vi "Start Search Params.vi"(8 "error in (no error)":errorcluster, 10 "Search in":refnum<class "Search.lvclass">, 11 "BetterSearch in":refnum<class "BetterSearch.lvclass">) -> (0 "error out":errorcluster, 2 "Start Params":T1, 3 "BetterSearch out":refnum<class "BetterSearch.lvclass">)   [LabVIEW 2020, in "Better Search.lvlib" / "BetterSearch.lvclass"]
uses:
  BetterSearch.lvclass
  Data Types/Search Params.ctl
  Data Types/Search Type.ctl
  Data Types/Search Scope.ctl
  Data Types/Scope Options.ctl
  Search/Search.lvclass
  BetterSearch.lvclass/BetterSearch.ctl
  Better Search.lvlib
panel:
  # "Exclude"
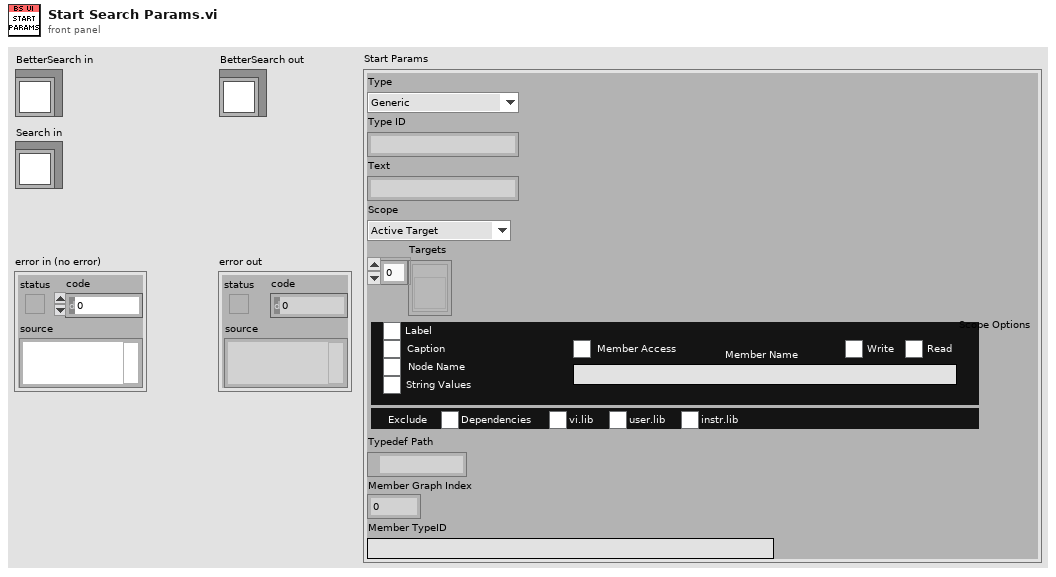
[diagram p1: front panel]
types:
  T1 = typedef "Better Search.lvlib/Search Params.ctl" = cluster{"Type":T2, "Type ID":string, "Text":string, "Scope":T3, "Targets":refnum<vi>[], "Scope Options":T4, "Typedef Path":path, "Member Graph Index":i32, "Member TypeID":string}
  T2 = typedef "Better Search.lvlib/Search Type.ctl" = enum16{"Generic", "Text", "Data Type", "VI", "Node"}
  T3 = typedef "Better Search.lvlib/Search Scope.ctl" = enum16{"Active Target", "Active Project", "Specific Targets", "Active VI", "Active Hierarchy"}
  T4 = typedef "Better Search.lvlib/Scope Options.ctl" = cluster{"Include Labels":bool, "Include Captions":bool, "Include Node Name":bool, "Member Access":bool, "Member Read":bool, "Member Write":bool, "Member Name":string, "String Value":bool, "Dependencies":bool, "vi.lib":bool, "user.lib":bool, "instr.lib":bool}
  T5 = typedef "Better Search.lvlib/Search Context.ctl" = cluster{"Type ID":string, "VI Refnum":refnum<vi>, "Starting Text":string, "Shift?":bool, "App Ref":refnum<vi>, "Start Search Type":T6, "Item Graph":T7[], "Variant":variant}
  T6 = typedef "Better Search.lvlib/Start Search Type.ctl" = enum16{"Auto", "Text", "Data Type", "Bundle"}
  T7 = typedef "Better Search.lvlib/Type Reflection Item.ctl" = cluster{"Parent":i32, "Depth":i32, "Children":i32[], "Skip":bool, "Name":string, "Type":variant, "TypeID":string}
  T8 = typedef "Better Search.lvlib/Search Type Info.ctl" = cluster{"Search Type":T2, "Name":string, "Item":variant}
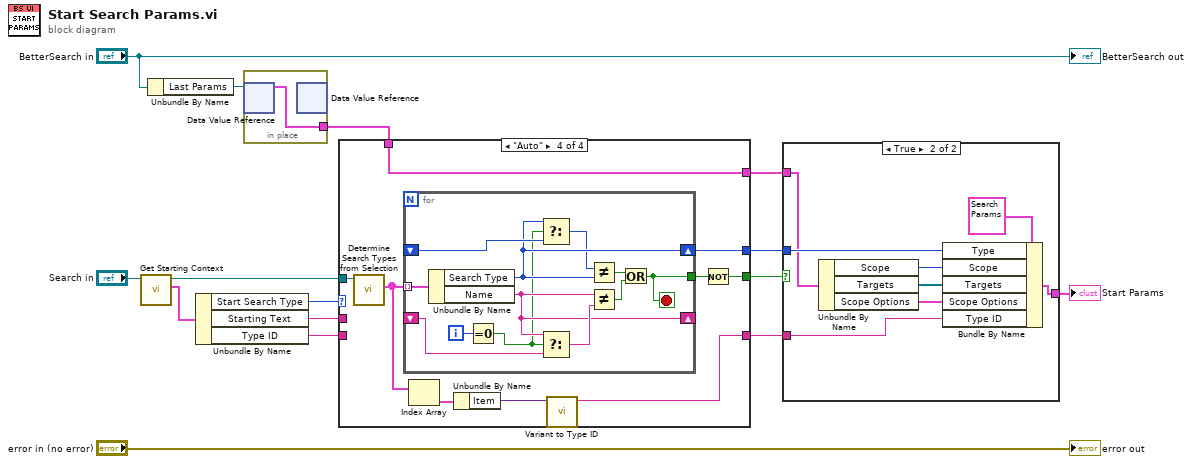
[diagram p0: block diagram]
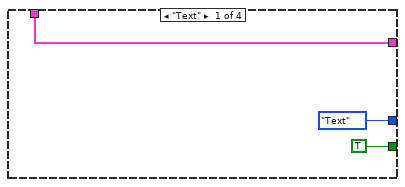
[diagram p2: hidden frame]
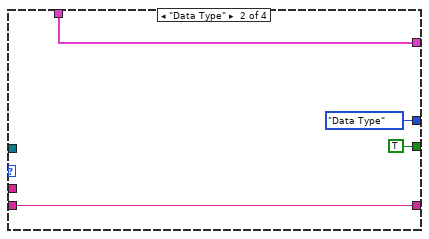
[diagram p3: hidden frame]
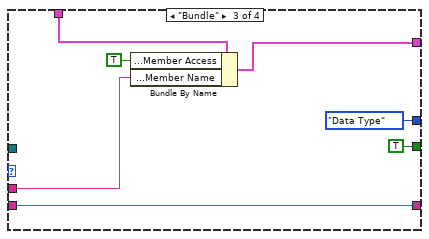
[diagram p4: hidden frame]
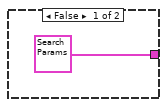
[diagram p5: hidden frame]
diagram:
  n1 = call "Get Starting Context.vi"("Search in"="Search in") -> ("Starting Context"=w7:T5, "Search out"=w8:refnum<class "Search.lvclass">)  [unwired: 8 in, 1 out]
  n2 = Unbundle By Name("BetterSearch in") -> ("Last Params"=w11:refnum<data-value>)
  n3 = Unbundle By Name(w7) -> ("Start Search Type"=w5:T6, "Starting Text"=w4:string, "Type ID"=w3:string)
  n4 = in-place {
    in-place-border: [w16] -> w2
    n5 = in-place-dvr #1(w11) -> (w16:T1)  [unwired: 1 out]
    n6 = in-place-dvr #1() -> ()  [unwired: 1 in, 2 out]
  }
  n7 = case shown="\"Auto\"" w5 {
    tunnel: [TRUE TRUE TRUE w34] -> w14
    tunnel: [Search_Type."Text" ("Search Type") Search_Type."Data Type" ("Search Type") Search_Type."Data Type" ("Search Type") w38] -> w13
    tunnel: w8 -> [_ _ _ w37]
    tunnel: [_ w21 w30 w31] -> w6
    tunnel: w4 -> [_ _ w26 _]
    tunnel: w3 -> [_ w21 w30 _]
    tunnel: w2 -> [w17 w20 w29 w33]
    tunnel: [w17 w20 w27 w33] -> w1
    frame "Text" {
    }
    frame "Data Type" {
    }
    frame "Bundle" {
      n8 = Bundle By Name(cluster=w29, "Scope Options.Member Access"=TRUE, "Scope Options.Member Name"=w26) -> (w27:T1)
    }
    frame "Auto" {
      n9 = call "Determine Search Types from Selection.vi"("Search in"=w37) -> ("Search Type Infos"=w35:T8[])  [unwired: 8 in, 2 out]
      n10 = for {
        tunnel: w35 -> [w51] mode=indexing
        shift-right: [w48] -> w38
        shift-left: _ -> [w49]
        shift-right: [w45] -> _
        shift-left: _ -> [w44]
        tunnel: [w40] -> w39
        i -> [w50]
        stop <- w40 stop-if-true
        n11 = Unbundle By Name(w51) -> ("Search Type"=w48:T2, "Name"=w45:string)
        n12 = Equal To 0?(x=w50) -> (x = 0?=w41:bool)
        n13 = Select(t=w48, s=w41, f=w49) -> (s? t:f=w47:T2)
        n14 = Select(t=w45, s=w41, f=w44) -> (s? t:f=w46:string)
        n15 = Not Equal?(x=w47, y=w48) -> (x != y?=w43:bool)
        n16 = Not Equal?(x=w45, y=w46) -> (x != y?=w42:bool)
        n17 = Or(x=w43, y=w42) -> (x .or. y?=w40:bool)
      }
      n18 = Index Array(array=w35) -> (element=w36:T8)  [unwired: 1 in]
      n19 = Unbundle By Name(w36) -> ("Item"=w32:variant)
      n20 = call "Variant to Type ID.vi"("Variant"=w32) -> ("Type ID"=w31:string)  [unwired: 9 in, 1 out]
      n21 = Not(x=w39) -> (.not. x?=w34:bool)
    }
  }
  n22 = case shown="True" w14 {
    tunnel: w13 -> [_ w58]
    tunnel: [T1 {"Type"=enum."Generic", "Type ID"="", "Text"="", "Scope"=enum."Active Target", "Targets"=[], "Scope Options"={"Include Labels"=FALSE, "Include Captions"=FALSE, "Include Node Name"=FALSE, "Member Access"=FALSE, "Member Read"=FALSE, "Member Write"=FALSE, "Member Name"="", "String Value"=FALSE, "Dependencies"=FALSE, "vi.lib"=FALSE, "user.lib"=FALSE, "instr.lib"=FALSE}, "Typedef Path"=path "", "Member Graph Index"=0, "Member TypeID"=""} ("Start Params") w59] -> w12
    tunnel: w6 -> [_ w54]
    tunnel: w1 -> [_ w53]
    frame False {
    }
    frame True {
      n23 = Unbundle By Name(w53) -> ("Scope"=w57:T3, "Targets"=w56:refnum<vi>[], "Scope Options"=w55:T4)
      n24 = Bundle By Name(cluster=T1 {"Type"=enum."Generic", "Type ID"="", "Text"="", "Scope"=enum."Active Target", "Targets"=[], "Scope Options"={"Include Labels"=FALSE, "Include Captions"=FALSE, "Include Node Name"=FALSE, "Member Access"=FALSE, "Member Read"=FALSE, "Member Write"=FALSE, "Member Name"="", "String Value"=FALSE, "Dependencies"=FALSE, "vi.lib"=FALSE, "user.lib"=FALSE, "instr.lib"=FALSE}, "Typedef Path"=path "", "Member Graph Index"=0, "Member TypeID"=""} ("Start Params"), "Type"=w58, "Scope"=w57, "Targets"=w56, "Scope Options"=w55, "Type ID"=w54) -> (w59:T1)
    }
  }
  "Start Params" <- w12
  "error out" <- "error in (no error)"
  "BetterSearch out" <- "BetterSearch in"
